vi "S2C_UNITHERM_Proc_Write-Read.vi"(7 "Local?":bool, 8 "Error In":errorcluster, 10 "Return":string, 11 "Command":string) -> (0 "Error Out":errorcluster, 3 "Response":variant)   [LabVIEW 2024]
uses:
  S2C_UNITHERM_Proc_Globals.vi
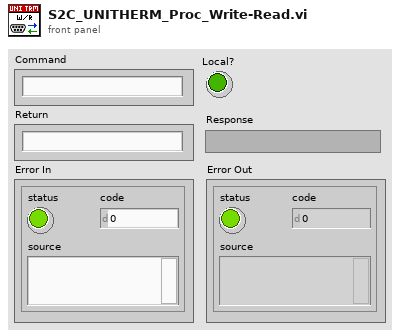
[diagram p1: front panel]
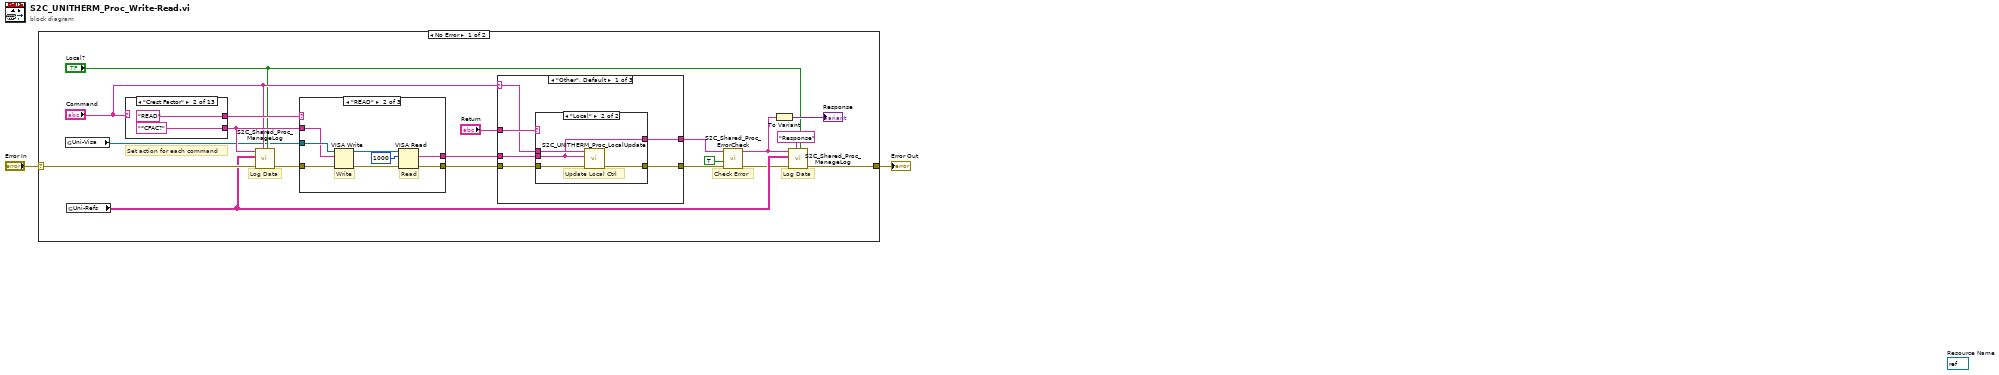
[diagram p0: block diagram]
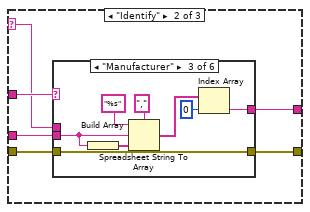
[diagram p3: hidden frame]
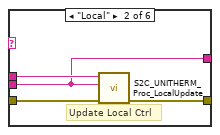
[diagram p5: hidden frame]
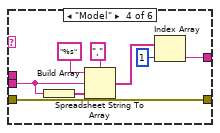
[diagram p6: hidden frame]
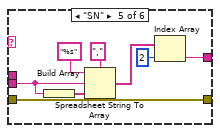
[diagram p7: hidden frame]
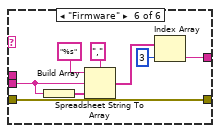
[diagram p8: hidden frame]
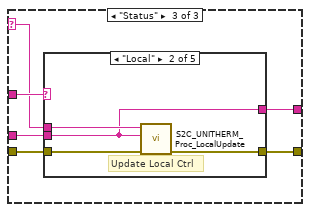
[diagram p9: hidden frame]
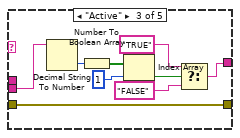
[diagram p11: hidden frame]
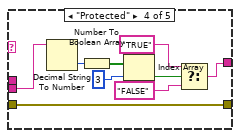
[diagram p12: hidden frame]
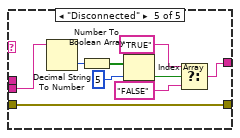
[diagram p13: hidden frame]
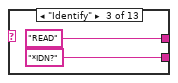
[diagram p15: hidden frame]
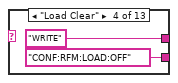
[diagram p16: hidden frame]
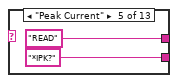
[diagram p17: hidden frame]
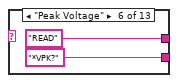
[diagram p18: hidden frame]
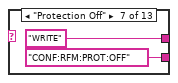
[diagram p19: hidden frame]
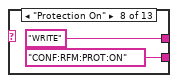
[diagram p20: hidden frame]
diagram:
  (unwired) refnum<visa-resource-name> refnum  # Resource Name
  n1 = case shown="No Error" "Error In" {
    selector: "Error In" -> [w16 w154]
    tunnel: [w13 w154] -> w1
    frame No Error {
      # "Check Error"
      # "Set action for each command"
      # "Log Data"
      # "Log Data"
      n2 = global read "S2C_UNITHERM_Proc_Globals.vi" "Uni-Visa"() -> (w3:refnum<visa-resource-name>)
      n3 = global read "S2C_UNITHERM_Proc_Globals.vi" "Uni-Refs"() -> (w9:string[][])
      n4 = case shown="\"Crest Factor\"" "Command" {
        tunnel: [_ "READ" "READ" "WRITE" "READ" "READ" "WRITE" "WRITE" "WRITE" "READ" "READ" "READ" "READ"] -> w20
        tunnel: [_ "*CFAC?" "*IDN?" "CONF:RFM:LOAD:OFF" "*IPK?" "*VPK?" "CONF:RFM:PROT:OFF" "CONF:RFM:PROT:ON" "*RST" "*IRMS?" "*VRMS?" "*TST?" "STAT?"] -> w14
        frame "Other", Default {
        }
        frame "Crest Factor" {
        }
        frame "Identify" {
        }
        frame "Load Clear" {
        }
        frame "Peak Current" {
        }
        frame "Peak Voltage" {
        }
        frame "Protection Off" {
        }
        frame "Protection On" {
        }
        frame "Reset" {
        }
        frame "RMS Current" {
        }
        frame "RMS Voltage" {
        }
        frame "SelfTest" {
        }
        frame "Status" {
        }
      }
      n5 = call "S2C_Shared_Proc_ManageLog.vi"("Local?"="Local?", "Command"="Command", "Error In"=w16, "Refs"=w9, "Data In"=w14) -> ("Error Out"=w15:errorcluster)  [unwired: 5 in, 1 out]
      n6 = case shown="\"READ\"" w20 {
        tunnel: [w140 w145 w151] -> w19
        tunnel: w15 -> [w140 w144 w153]
        tunnel: w3 -> [_ w143 w152]
        tunnel: ["Unknown" ("read buffer") w142 "Success" ("read buffer")] -> w18
        tunnel: w14 -> [_ w141 w150]
        frame "Other", Default {
        }
        frame "READ" {
          # "Read"
          # "Write"
          n7 = VISA Write(VISA resource name=w143, write buffer=w141, error in (no error)=w144) -> (VISA resource name out=w147:refnum<visa-resource-name>, error out=w148:errorcluster)  [unwired: 1 out]
          n8 = VISA Read(VISA resource name=w147, byte count=u32 1000, error in (no error)=w148) -> (read buffer=w142:string, error out=w145:errorcluster)  [unwired: 2 out]
        }
        frame "WRITE" {
          # "Write"
          n9 = VISA Write(VISA resource name=w152, write buffer=w150, error in (no error)=w153) -> (error out=w151:errorcluster)  [unwired: 2 out]
        }
      }
      n10 = case shown="\"Other\", Default" "Command" {
        selector: "Command" -> [w22 w34 w77]
        tunnel: w19 -> [w27 w39 w81]
        tunnel: w18 -> [w24 w38 w78]
        tunnel: "Return" -> [w26 w37 w79]
        tunnel: [w25 w36 w80] -> w7
        tunnel: [w23 w35 w82] -> w6
        frame "Other", Default {
          n11 = case shown="\"Local\"" w26 {
            tunnel: w27 -> [w29 w33]
            tunnel: [w29 w32] -> w25
            tunnel: w24 -> [w28 w30]
            tunnel: [w28 w30] -> w23
            tunnel: w22 -> [_ w31]
            frame "Other", Default {
            }
            frame "Local" {
              # "Update Local Ctrl"
              n12 = call "S2C_UNITHERM_Proc_LocalUpdate.vi"("Error In"=w33, "Data"=w30, "Command"=w31) -> ("Error Out"=w32:errorcluster)  [unwired: 8 in]
            }
          }
        }
        frame "Identify" {
          n13 = case shown="\"Manufacturer\"" w37 {
            tunnel: w39 -> [w40 w44 w52 w60 w68 w76]
            tunnel: w38 -> [_ w41 w49 w57 w65 w73]
            tunnel: [w40 w43 w52 w60 w68 w76] -> w36
            tunnel: [_ w41 w45 w53 w61 w69] -> w35
            tunnel: w34 -> [_ w42 _ _ _ _]
            frame "Other", Default {
            }
            frame "Local" {
              # "Update Local Ctrl"
              n14 = call "S2C_UNITHERM_Proc_LocalUpdate.vi"("Error In"=w44, "Data"=w41, "Command"=w42) -> ("Error Out"=w43:errorcluster)  [unwired: 8 in]
            }
            frame "Manufacturer" {
              n15 = Build Array(w49) -> (w48:string[])
              n16 = Spreadsheet String To Array(delimiter (Tab)=",", format string="%s", spreadsheet string=w49, array type (2D Dbl)=w48) -> (array=w47:string[])
              n17 = Index Array(array=w47, index=0) -> (element=w45:string)
            }
            frame "Model" {
              n18 = Build Array(w57) -> (w56:string[])
              n19 = Spreadsheet String To Array(delimiter (Tab)=",", format string="%s", spreadsheet string=w57, array type (2D Dbl)=w56) -> (array=w55:string[])
              n20 = Index Array(array=w55, index=1) -> (element=w53:string)
            }
            frame "SN" {
              n21 = Build Array(w65) -> (w64:string[])
              n22 = Spreadsheet String To Array(delimiter (Tab)=",", format string="%s", spreadsheet string=w65, array type (2D Dbl)=w64) -> (array=w63:string[])
              n23 = Index Array(array=w63, index=2) -> (element=w61:string)
            }
            frame "Firmware" {
              n24 = Build Array(w73) -> (w72:string[])
              n25 = Spreadsheet String To Array(delimiter (Tab)=",", format string="%s", spreadsheet string=w73, array type (2D Dbl)=w72) -> (array=w71:string[])
              n26 = Index Array(array=w71, index=3) -> (element=w69:string)
            }
          }
        }
        frame "Status" {
          n27 = case shown="\"Local\"" w79 {
            tunnel: [_ w84 w91 w100 w109] -> w82
            tunnel: w81 -> [w83 w87 w89 w98 w107]
            tunnel: [w83 w86 w89 w98 w107] -> w80
            tunnel: w78 -> [_ w84 w88 w97 w106]
            tunnel: w77 -> [_ w85 _ _ _]
            frame "Other", Default {
            }
            frame "Local" {
              # "Update Local Ctrl"
              n28 = call "S2C_UNITHERM_Proc_LocalUpdate.vi"("Error In"=w87, "Data"=w84, "Command"=w85) -> ("Error Out"=w86:errorcluster)  [unwired: 8 in]
            }
            frame "Active" {
              n29 = Decimal String To Number(string=w88) -> (number=w96:i32)  [unwired: 2 in, 1 out]
              n30 = Number To Boolean Array(number=w96) -> (Boolean array=w95:bool[])
              n31 = Index Array(array=w95, index=1) -> (element=w93:bool)
              n32 = Select(t="TRUE", s=w93, f="FALSE") -> (s? t:f=w91:string)
            }
            frame "Protected" {
              n33 = Decimal String To Number(string=w97) -> (number=w105:i32)  [unwired: 2 in, 1 out]
              n34 = Number To Boolean Array(number=w105) -> (Boolean array=w104:bool[])
              n35 = Index Array(array=w104, index=3) -> (element=w102:bool)
              n36 = Select(t="TRUE", s=w102, f="FALSE") -> (s? t:f=w100:string)
            }
            frame "Disconnected" {
              n37 = Decimal String To Number(string=w106) -> (number=w114:i32)  [unwired: 2 in, 1 out]
              n38 = Number To Boolean Array(number=w114) -> (Boolean array=w113:bool[])
              n39 = Index Array(array=w113, index=5) -> (element=w111:bool)
              n40 = Select(t="TRUE", s=w111, f="FALSE") -> (s? t:f=w109:string)
            }
          }
        }
      }
      n41 = call "S2C_Shared_Proc_ErrorCheck.vi"("Error In"=w7, "ExpReply?"=TRUE, "Reply Text"=w6) -> ("Error Out"=w8:errorcluster, "Status"=w5:string)  [unwired: 7 in]
      n42 = To Variant(anything=w5) -> (Variant=→"Response":variant)
      n43 = call "S2C_Shared_Proc_ManageLog.vi"("Local?"="Local?", "Command"="Response", "Error In"=w8, "Refs"=w9, "Data In"=w5) -> ("Error Out"=w13:errorcluster)  [unwired: 5 in, 1 out]
    }
    frame Error {
    }
  }
  "Error Out" <- w1
